vi "Setting Database Name.vi"(9 "error in (no error)":errorcluster) -> (1 "error out":errorcluster, 3 "Name":string="Object Settings Database")   [LabVIEW 2019, in "Setting Database.lvclass"]
uses:
  Setting Database.lvclass
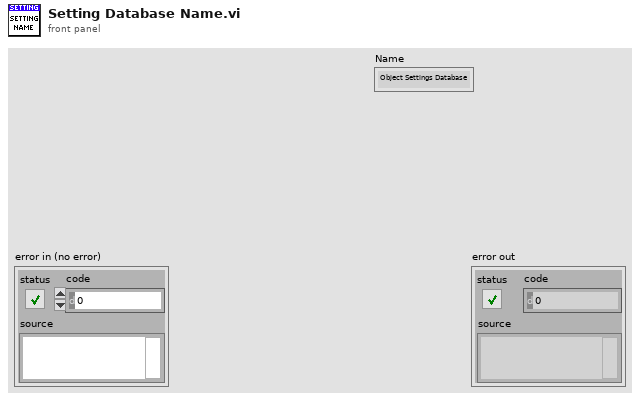
[diagram p1: front panel]
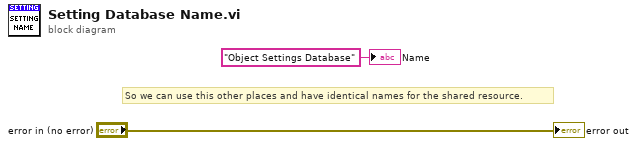
[diagram p0: block diagram]
diagram:
  # "So we can use this other places and have identical names for the shared resource."
  "Name" <- "Object Settings Database"
  "error out" <- "error in (no error)"
